vi "Autonomous Independent.vi"() -> ()   [LabVIEW 2015]
doc: "If AutoIDs match then TwoBall? is read from Dashboard, Else it is a control on the Front Panel\n\nINPUTS:\nTwoBall?\nState (Init)\nCollectorArmSpeed\nBrakeDistance\nSlowdownDistance\n\nSTATES:\n\nINIT: Clapper - In, SonicShifter Actuates to Low Gear, RollerPnuematic - Out, Servo - SetAngle (Indicator on Front Panel), IF TwoBall? == True: LowerArm ELSE CheckHotGoal\n\nCHECKHOTGOAL: Runs IsHotGoalDB and puts HotGoal? into Shift Register\n\nLOWERARM: Clapper - OUT, Wait = LowerArmTimeout / 2, RollerPneumatic - WAIT, Collector- LOWER\nWhen Collector has finished or after timeout from LowerArmTimeout and two other timers, Collector - STOP\nIF TwoBall? == TRUE then Collect ELSE Drive12ft\n\nPRECOLLECT: CollectorWrapper - PRECOLLECT\n\nDRIVEBACK: TankDrive -SETVALUE and DriveBackSpeed goes into both desired speeds, Wait - DriveBackWait, TankDrive - SETVALUE and 0 for both desired speeds\n\nCOLLECT: CollectWrapper - COLLECT\n\nSTOPCOLLECT: CollectWrapper - STOP\n\nLIFTARM: Collector - RAISE, Wait - LiftArmWait, Collector - STOP\n\nRAISESERVO: Servo - SETANGLE, Servo takes in RaiseServoAngle from Front Panel\n\nDRIVE12FT: Sonar - READVALUE, AutoDistance - LINEAR, Takes in Drive12ftDistance and distance from the Sonar and BrakeDistance and SlowdownDistance, TankDrive - LINEARDRIVE, Takes in both motor values from AutoDistance and MaxMotorChangeForward/Backward for Desired, TankDrive - LINEARDRIVE, Takes in 0 for Desired and MaxMotorChanges\n\nSHOOT12FT: IF not TwoBall? AND not HotGoal? then Wait - 5500 - ElapsedTime ELSE Pass, Wait - PreShootWait, ShooterWrapper - COLLECTORDOWN\n\nRAISEARM: Wait - PreRaiseArmWait, Collector - RAISE, Takes in CollectorArmSpeed, After Timeout from RaiseArmTimeout or Collector is done , Collector - STOP\n\nSHOOT3FT: Sonar - READVALUE, AutoDistance - LINEAR, Takes in Drive3ftDistance and output form Sonar and Brake/SlowdownDistance, TankDrive - SETVALUE, Takes in AutoDistance values for desired, Exits after AutoDistance is done or Drive3tfTimeout, TankDrive - SETVALUE, Takes in 0 for desired\n\nSHOOT3FT: ShooterWrapper - COLLECTORUP\n\nSTOP: Servo - SETANGLE, 0 for angle"
uses:
  AutoStates.ctl
  Robot Global Data.vi
  SingleSolenoidAction.ctl
  DoubleSolenoidAction.ctl
  ServoAction.ctl
  CollectorAction.ctl
  CollectorWrapAction.ctl
  TankDriveAction.ctl
  AutoAlignMode.ctl
  SonarAction.ctl
  ShooterWrapperAction.ctl
  AutoMode.ctl
  RollerAction.ctl
  LEDSaction.ctl
  HotGoalDetectType.ctl
panel:
  in  "PreScumbagWait":u32
  in  "HotGoalTypeDefault":T1
  out "KinectTriggered?":bool
  in  "EndInLowGear?":bool=TRUE
  in  "DriveBackWait":u32=1000
  in  "DriveBackSpeed":dbl=-1.0
  in  "PreCheckGoalWait":u32=260
  in  "BallSettleWait":u32=130
  in  "StartShootTime":u32=5000
  in  "StartInLowGear?":bool=TRUE
  in  "PreCollectWait":u32=400
  in  "AutoIDKey":i32=3061
  in  "DefaultMotorInput":dbl=1.0
  in  "DriveMinTime":u32=2000
  in  "RotateWait":u32=300
  in  "RotateMotorInput":dbl=0.7
  in  "DriveDistance":dbl=36.0 format="%#_13g"
  in  "DriveTimeout":u32=4000
  out "CheckGoalTimedOut?":bool
  in  "CheckHotGoalTimeout":u32=800
  in  "AutoDefaultMode":T2
  in  "ServoInitAngle":i32=140
  in  "RaiseServoAngle":i32=100
  in  "AccelBackward":dbl=0.1
  in  "PreRaiseArmWait":u32=500
  in  "AccelForward":dbl=0.1
  out "ElapsedTime":u32
  out "StateTime":u32
  out "CurrentState":T3
  out "RaiseArmTimedOut":bool
  out "Hot?":bool
  out "DriveTimeOut":bool
  out "LowerArmTimedOut":bool
  in  "RaiseArmTimeout":u32=800
  in  "SlowdownDistance":dbl=36.0 format="%#_13g"
  in  "BrakeDistance":dbl=12.0 format="%#_13g"
  in  "CollectorArmSpeed":dbl=1.0 format="%#_13g"
  in  "LiftArmWait":u32=200
  in  "PreDriveBackWait":u32
  in  "PreDriveBackSpeed":dbl
  in  "LowerArmTimeout":u32=800
  in  "error in":errorcluster
  out "error out":errorcluster
  # "SHOOT"
  # "SERVO"
  # "HOT GOAL"
  # "OUTPUT"
  # "ROTATE"
  # "GENERAL"
  # "DRIVE"
  # "RAISE/LOWER ARM"
  # "DEPRECATED"
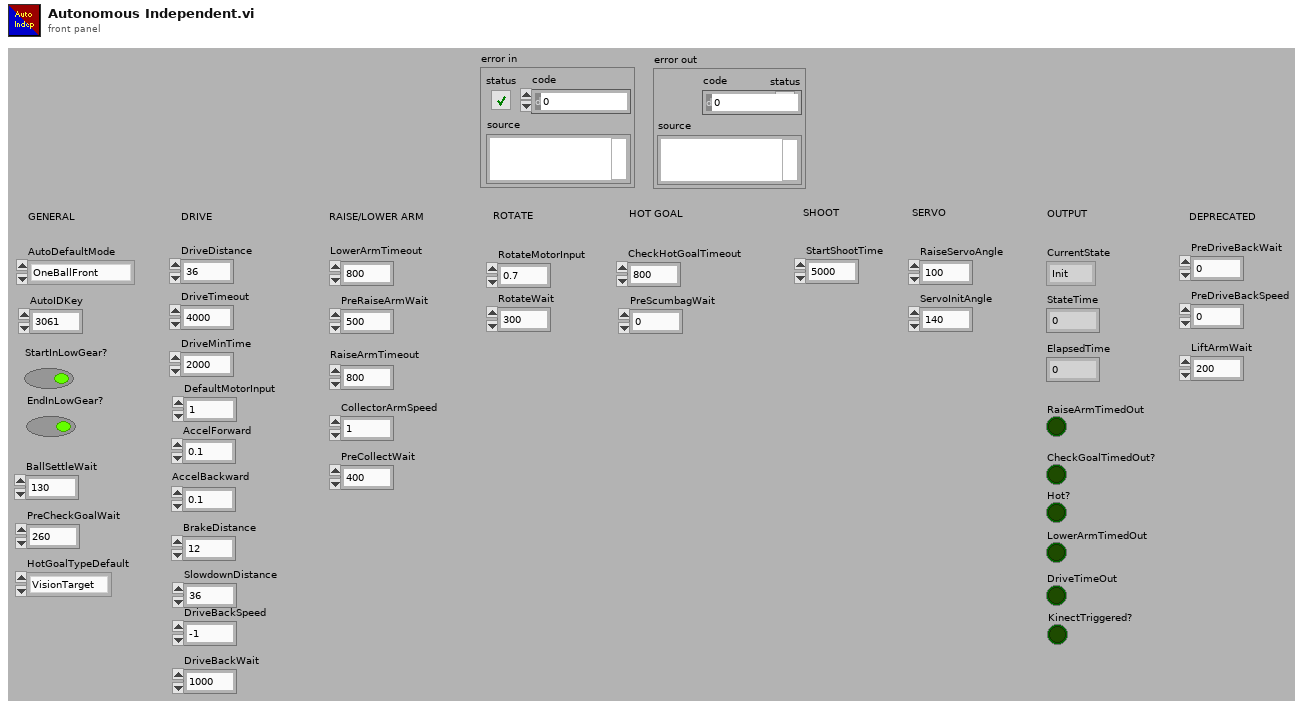
[diagram p1: front panel]
types:
  T1 = typedef "HotGoalDetectType.ctl" = enum16{"VisionTarget", "Kinect", "SoundDetect", "Webcam"}
  T2 = typedef "AutoMode.ctl" = enum16{"OneBallFront", "OneBallCollector", "TwoBallNormal", "TwoBallHot"}
  T3 = typedef "AutoStates.ctl" = enum16{"Init", "LowerArmCheckGoal", "DriveBack", "Collect", "StopCollect", "LiftArm", "RaiseServo", "Drive", "ShootCollectorUp", "RaiseArm", "ShootCollectorDown", "Rotate1", "Rotate2", "Stop"}
  T4 = typedef "SingleSolenoidAction.ctl" = enum16{"Init", "SetState", "Disable"}
  T5 = typedef "DoubleSolenoidAction.ctl" = enum16{"Init", "Middle", "In", "Out"}
  T6 = typedef "ServoAction.ctl" = enum16{"Init", "SetAngle", "GetAngle", "Lower", "Raise", "Disable"}
  T7 = typedef "CollectorAction.ctl" = enum16{"Init", "Raise", "Lower", "Stop", "GetStatus"}
  T8 = typedef "RollerAction.ctl" = enum16{"Init", "Off", "Forward", "Reverse"}
  T9 = typedef "TankDriveAction.ctl" = enum16{"Init", "LinearDrive", "SetValue", "Disable"}
  T10 = typedef "CollectorWrapAction.ctl" = enum16{"Stop", "PreCollect", "Collect"}
  T11 = typedef "AutoAlignMode.ctl" = enum16{"Fullspeed", "Linear"}
  T12 = typedef "SonarAction.ctl" = enum16{"Init", "ReadValue", "Disable"}
  T13 = typedef "LEDSaction.ctl" = enum16{"Init", "10SecondsLeft", "LimitDown", "LimitUp", "CollectDown", "CollectUp", "NotHot", "Hot", "Shift", "RollBack", "RollFwd", "Shoot", "Distance Low", "DistanceHigh", "PressureLow", "PressureHigh"}
  T14 = typedef "ShooterWrapperAction.ctl" = enum16{"Init", "CollectorDown", "CollectorUp"}
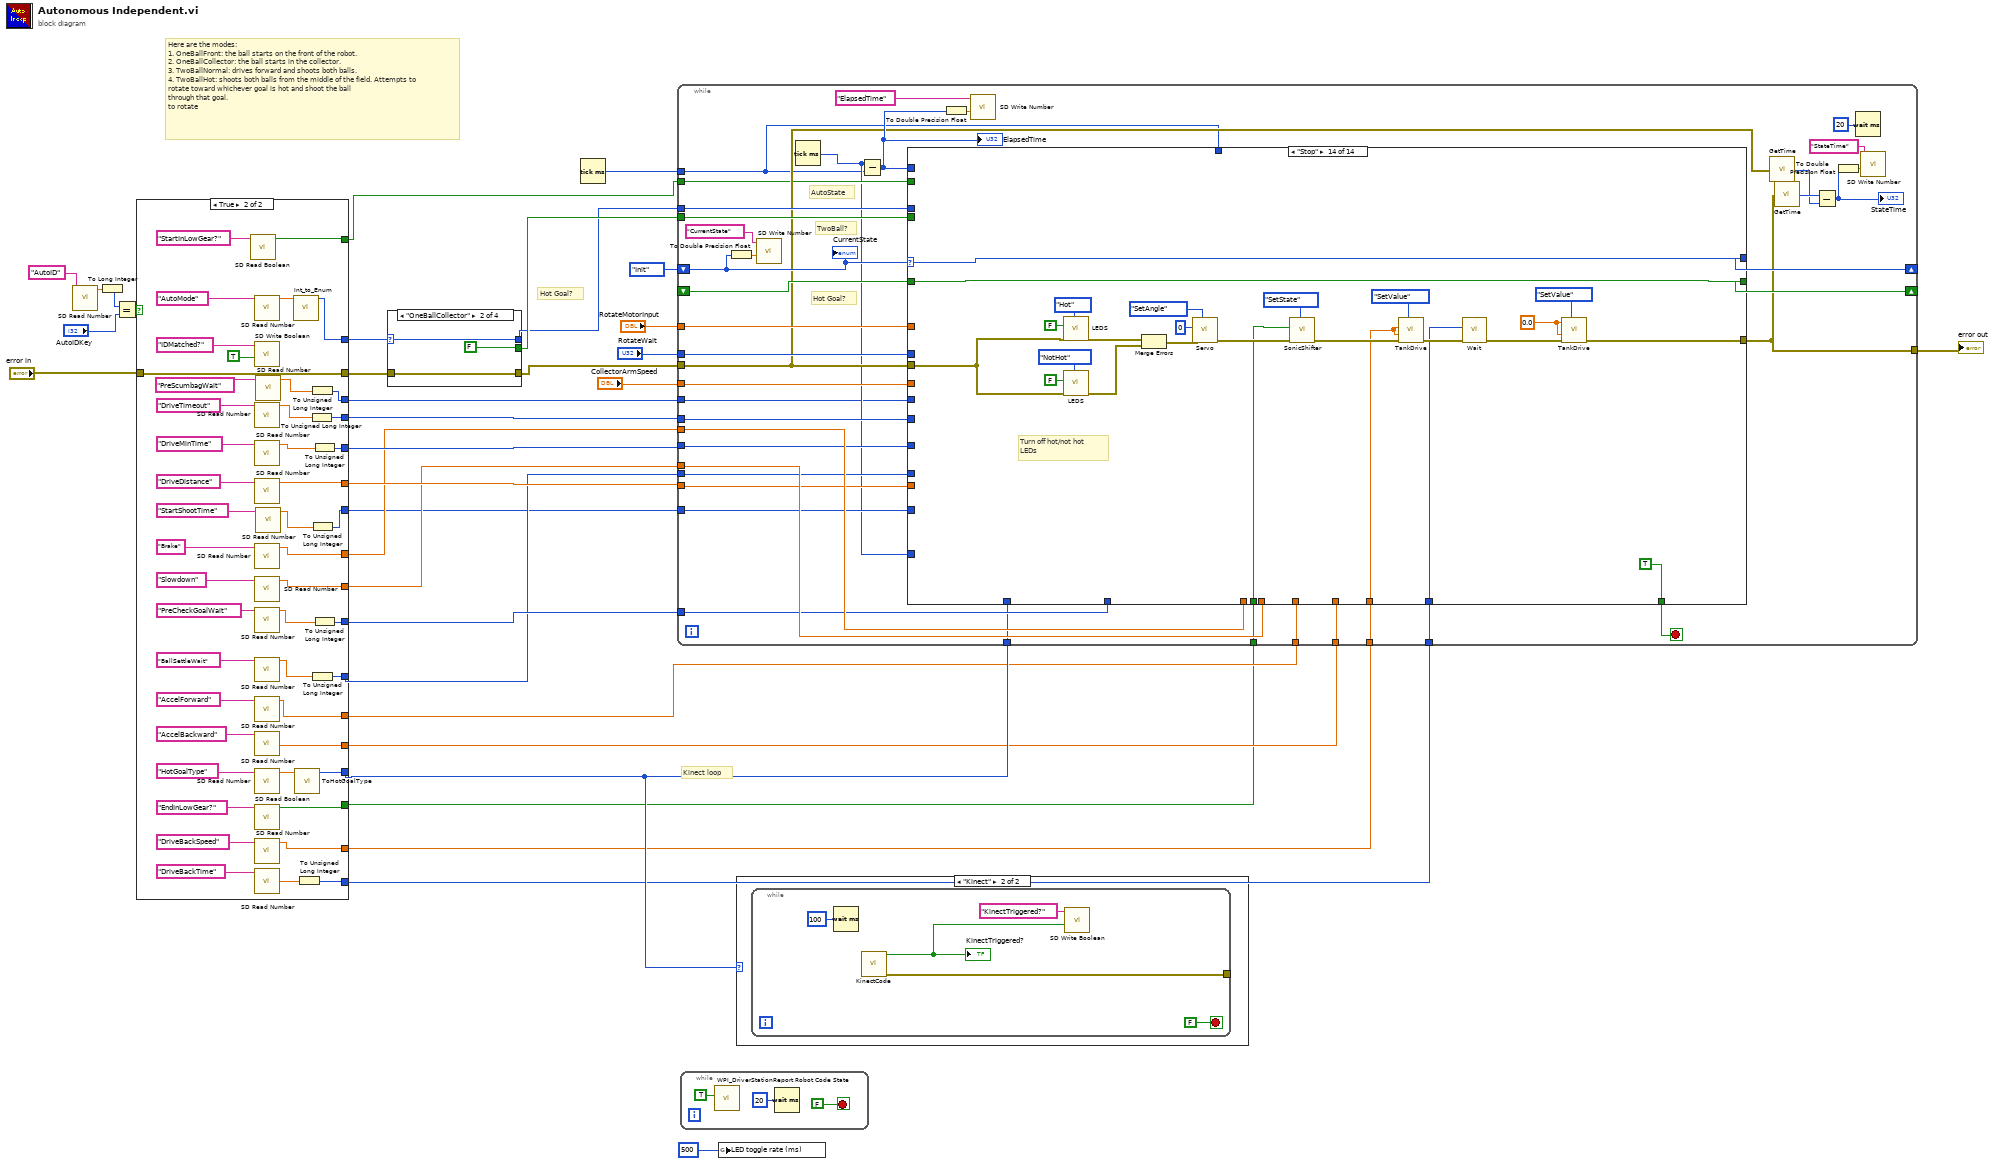
[diagram p0: block diagram]
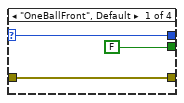
[diagram p3: hidden frame]
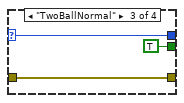
[diagram p4: hidden frame]
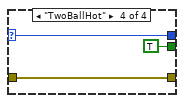
[diagram p5: hidden frame]
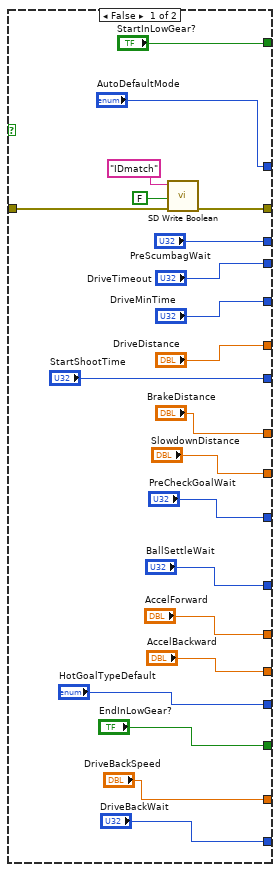
[diagram p6: hidden frame]
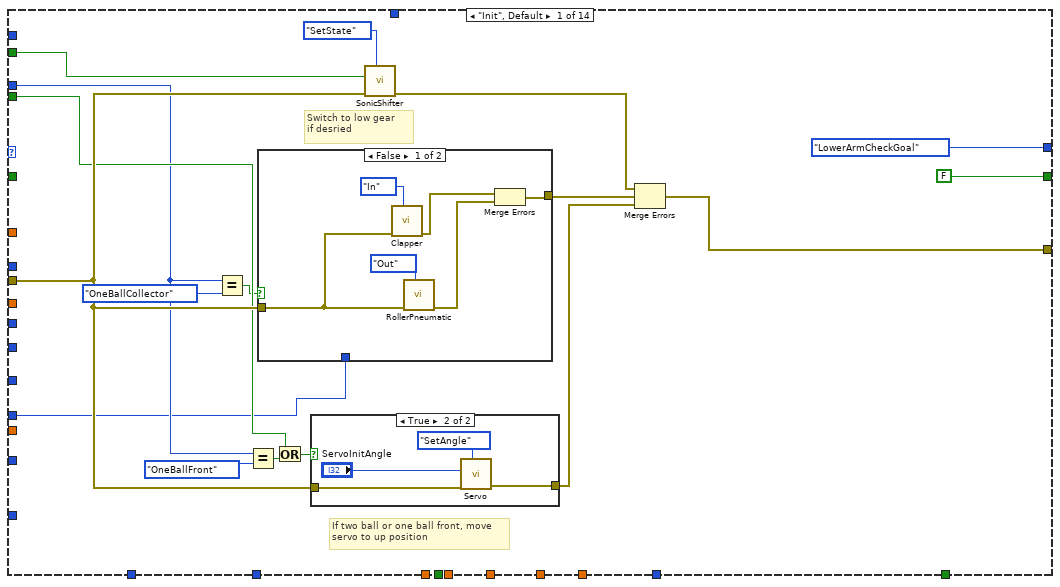
[diagram p7: hidden frame]
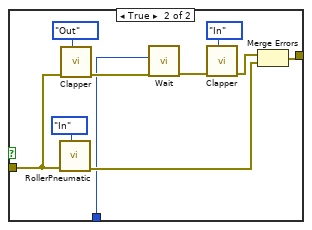
[diagram p8: hidden frame]
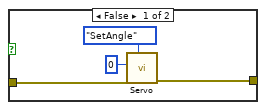
[diagram p9: hidden frame]
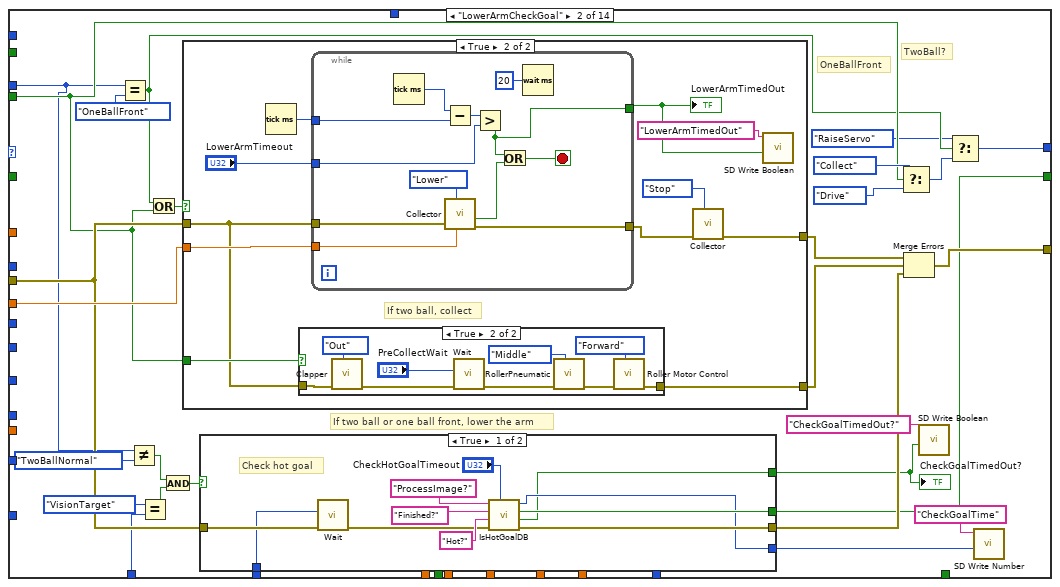
[diagram p10: hidden frame]
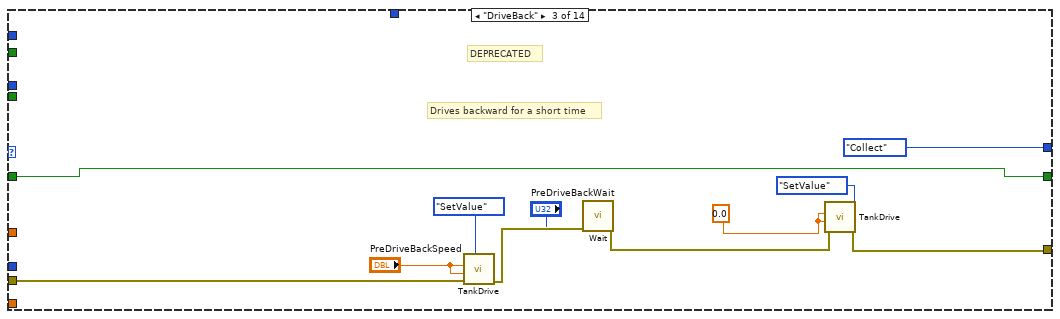
[diagram p14: hidden frame]
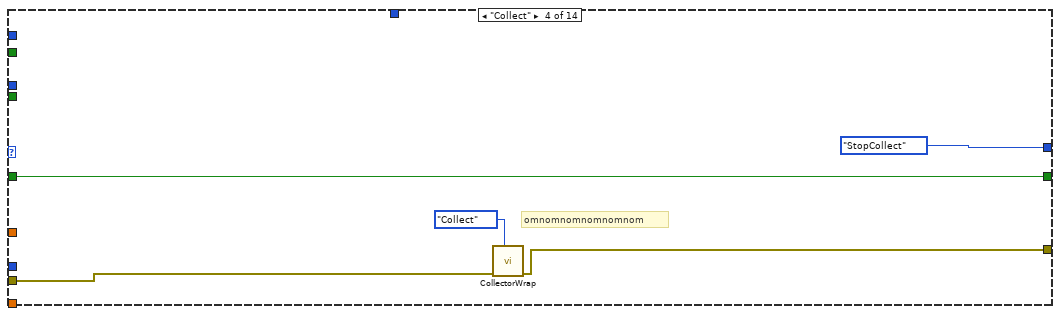
[diagram p15: hidden frame]
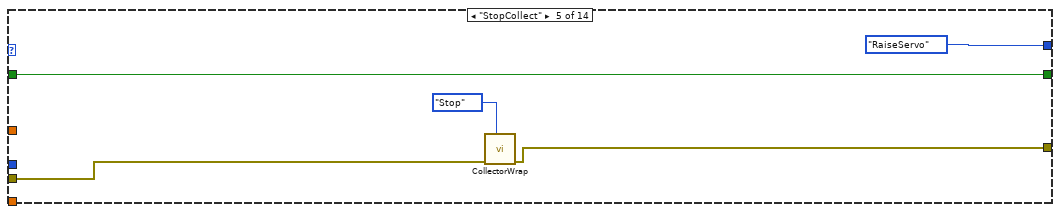
[diagram p16: hidden frame]
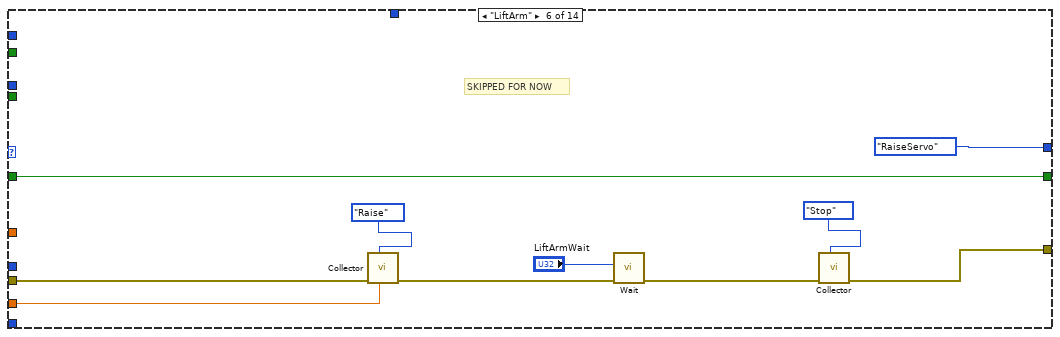
[diagram p17: hidden frame]
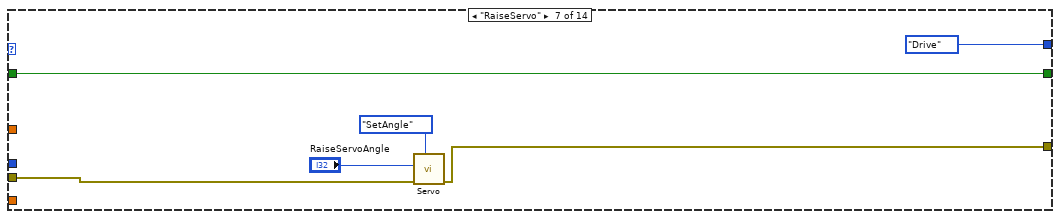
[diagram p18: hidden frame]
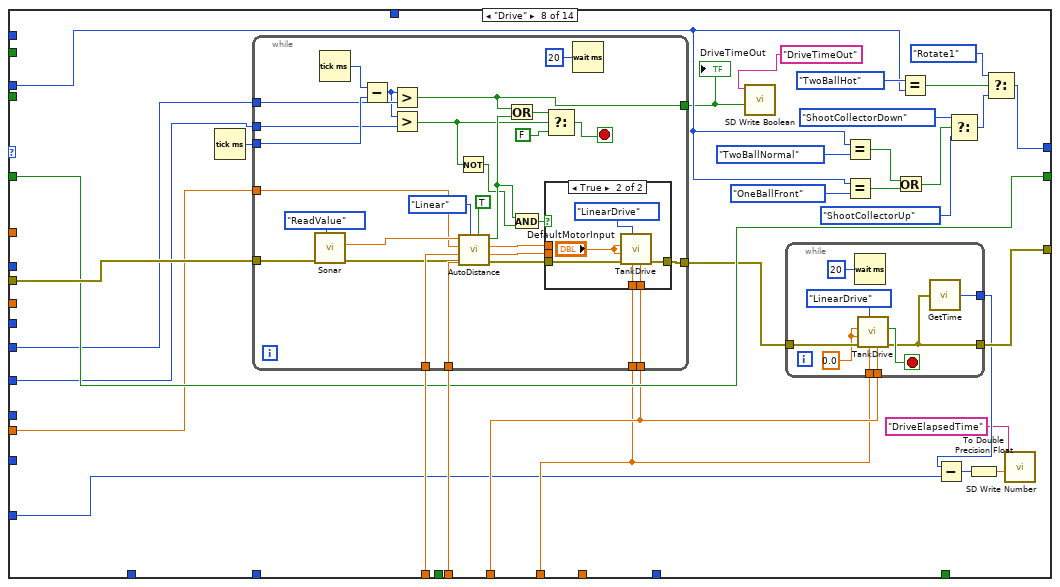
[diagram p19: hidden frame]
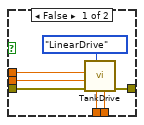
[diagram p20: hidden frame]
diagram:
  # "Kinect loop"
  # "Here are the modes:\n1. OneBallFront: the ball starts on the front of the robot.\n2. OneBallCollector: the ball starts in the collector.\n3. TwoBallNormal: drives forward and shoots both balls.\n4. TwoBallHot: shoots both balls from the middle of the field. Attempts to rotate toward whichever goal is hot and shoot the ball\nthrough that goal.\nto rotate"
  # "Hot Goal?"
  n1 = call <vilib>:"SD Read Number.vi"("Name"="AutoID") -> ("Numeric"=w33:dbl)  [unwired: 8 in, 2 out]
  n2 = To Long Integer(number=w33) -> (32bit integer=w19:i32)
  n3 = Equal?(x=w19, y="AutoIDKey") -> (x = y?=w28:bool)
  n4 = case shown="True" w28 {
    tunnel: "error in" -> [w54 w62]
    tunnel: [w53 w62] -> w24
    tunnel: ["AutoDefaultMode" w98] -> w26
    tunnel: ["DriveTimeout" w93] -> w14
    tunnel: ["DriveMinTime" w91] -> w15
    tunnel: ["DriveDistance" w89] -> w16
    tunnel: ["BrakeDistance" w87] -> w13
    tunnel: ["SlowdownDistance" w86] -> w12
    tunnel: ["PreCheckGoalWait" w83] -> w11
    tunnel: ["BallSettleWait" w80] -> w10
    tunnel: ["HotGoalTypeDefault" w76] -> w9
    tunnel: ["StartInLowGear?" w75] -> w8
    tunnel: ["AccelForward" w71] -> w7
    tunnel: ["AccelBackward" w70] -> w6
    tunnel: ["EndInLowGear?" w68] -> w5
    tunnel: ["DriveBackSpeed" w66] -> w4
    tunnel: ["DriveBackWait" w63] -> w3
    tunnel: ["StartShootTime" w59] -> w2
    tunnel: ["PreScumbagWait" w56] -> w1
    frame False {
      n5 = call <vilib>:"SD Write Boolean.vi"("error in"=w54, "Boolean"=FALSE, "Name"="IDmatch") -> ("error out"=w53:errorcluster)  [unwired: 7 in, 1 out]
    }
    frame True {
      n6 = call <vilib>:"SD Read Boolean.vi"("Name"="StartInLowGear?") -> ("Boolean"=w75:bool)  [unwired: 8 in, 2 out]
      n7 = call <vilib>:"SD Read Number.vi"("Name"="AutoMode") -> ("Numeric"=w99:dbl)  [unwired: 8 in, 2 out]
      n8 = call <vilib>:"SD Write Boolean.vi"("Boolean"=TRUE, "Name"="IDMatched?") -> ()  [unwired: 8 in, 2 out]
      n9 = call <vilib>:"SD Read Number.vi"("Name"="DriveTimeout") -> ("Numeric"=w92:dbl)  [unwired: 8 in, 2 out]
      n10 = call <vilib>:"SD Read Number.vi"("Name"="DriveMinTime") -> ("Numeric"=w90:dbl)  [unwired: 8 in, 2 out]
      n11 = call <vilib>:"SD Read Number.vi"("Name"="DriveDistance") -> ("Numeric"=w89:dbl)  [unwired: 8 in, 2 out]
      n12 = call <vilib>:"SD Read Number.vi"("Name"="Brake") -> ("Numeric"=w87:dbl)  [unwired: 8 in, 2 out]
      n13 = call <vilib>:"SD Read Number.vi"("Name"="Slowdown") -> ("Numeric"=w86:dbl)  [unwired: 8 in, 2 out]
      n14 = call <vilib>:"SD Read Number.vi"("Name"="PreCheckGoalWait") -> ("Numeric"=w82:dbl)  [unwired: 8 in, 2 out]
      n15 = call <vilib>:"SD Read Number.vi"("Name"="BallSettleWait") -> ("Numeric"=w79:dbl)  [unwired: 8 in, 2 out]
      n16 = call <vilib>:"SD Read Number.vi"("Name"="AccelForward") -> ("Numeric"=w71:dbl)  [unwired: 8 in, 2 out]
      n17 = call <vilib>:"SD Read Number.vi"("Name"="AccelBackward") -> ("Numeric"=w70:dbl)  [unwired: 8 in, 2 out]
      n18 = call <vilib>:"SD Read Number.vi"("Name"="HotGoalType") -> ("Numeric"=w77:dbl)  [unwired: 8 in, 2 out]
      n19 = call <vilib>:"SD Read Boolean.vi"("Name"="EndInLowGear?") -> ("Boolean"=w68:bool)  [unwired: 8 in, 2 out]
      n20 = call <vilib>:"SD Read Number.vi"("Name"="DriveBackSpeed") -> ("Numeric"=w66:dbl)  [unwired: 8 in, 2 out]
      n21 = call <vilib>:"SD Read Number.vi"("Name"="DriveBackTime") -> ("Numeric"=w65:dbl)  [unwired: 8 in, 2 out]
      n22 = call <vilib>:"SD Read Number.vi"("Name"="PreScumbagWait") -> ("Numeric"=w58:dbl)  [unwired: 8 in, 2 out]
      n23 = call <vilib>:"SD Read Number.vi"("Name"="StartShootTime") -> ("Numeric"=w61:dbl)  [unwired: 8 in, 2 out]
      n24 = call "Int_to_Enum.vi"("IntIn"=w99) -> ("EnumOut"=w98:T2)  [unwired: 10 in]
      n25 = call "ToHotGoalType.vi"("IntIn"=w77) -> ("EnumOut"=w76:T1)  [unwired: 10 in]
      n26 = To Unsigned Long Integer(number=w65) -> (unsigned 32bit integer=w63:u32)
      n27 = To Unsigned Long Integer(number=w92) -> (unsigned 32bit integer=w93:u32)
      n28 = To Unsigned Long Integer(number=w58) -> (unsigned 32bit integer=w56:u32)
      n29 = To Unsigned Long Integer(number=w79) -> (unsigned 32bit integer=w80:u32)
      n30 = To Unsigned Long Integer(number=w61) -> (unsigned 32bit integer=w59:u32)
      n31 = To Unsigned Long Integer(number=w90) -> (unsigned 32bit integer=w91:u32)
      n32 = To Unsigned Long Integer(number=w82) -> (unsigned 32bit integer=w83:u32)
    }
  }
  n33 = case shown="\"OneBallCollector\"" w26 {
    selector: w26 -> [w102 w105 w108 w111]
    tunnel: [FALSE FALSE TRUE TRUE] -> w25
    tunnel: w24 -> [w103 w106 w109 w112]
    tunnel: [w103 w106 w109 w112] -> w23
    tunnel: [w102 w105 w108 w111] -> w22
    frame "OneBallFront", Default {
    }
    frame "OneBallCollector" {
    }
    frame "TwoBallNormal" {
    }
    frame "TwoBallHot" {
    }
  }
  n34 = Tick Count (ms)() -> (millisecond timer value=w29:u32)
  n35 = while {
    shift-right: [w152] -> _
    shift-left: AutoStates."Init" ("Enum") -> [w134]
    shift-right: [w154] -> _
    shift-left: _ -> [w153]
    tunnel: w25 -> [w151]
    tunnel: "CollectorArmSpeed" -> [w149]
    tunnel: w13 -> [w147]
    tunnel: w12 -> [w148]
    tunnel: w29 -> [w114]
    tunnel: w23 -> [w131]
    tunnel: [w132] -> w34
    tunnel: w22 -> [w144]
    tunnel: "RotateMotorInput" -> [w143]
    tunnel: "RotateWait" -> [w142]
    tunnel: w2 -> [w129]
    tunnel: w16 -> [w128]
    tunnel: w15 -> [w127]
    tunnel: w14 -> [w126]
    tunnel: w11 -> [w125]
    tunnel: w10 -> [w124]
    tunnel: w9 -> [w123]
    tunnel: w8 -> [w122]
    tunnel: w7 -> [w121]
    tunnel: w6 -> [w120]
    tunnel: w5 -> [w118]
    tunnel: w4 -> [w117]
    tunnel: w3 -> [w116]
    tunnel: w1 -> [w115]
    stop <- w146 stop-if-true
    # "AutoState"
    # "TwoBall?"
    # "Hot Goal?"
    n36 = To Double Precision Float(number=w134) -> (double precision float=w135:dbl)
    n37 = call <vilib>:"SD Write Number.vi"("Numeric"=w135, "Name"="CurrentState") -> ()  [unwired: 8 in, 2 out]
    n38 = Tick Count (ms)() -> (millisecond timer value=w119:u32)
    n39 = Subtract(x=w119, y=w114) -> (x-y=w137:u32)
    "ElapsedTime" <- w137
    n40 = case shown="\"Stop\"" w134 {
      selector: w134 -> [_ _ _ _ _ _ _ _ _ _ _ _ _ w559]
      tunnel: w131 -> [w166 w221 w280 w285 w290 w295 w305 w337 w402 w465 w486 w509 w525 w541]
      tunnel: [w170 w220 w273 w284 w289 w294 w304 w334 w389 w463 w491 w504 w524 w547] -> w132
      tunnel: [FALSE ("Hot?") w208 w278 w282 w287 w293 w306 w326 w393 w464 w481 w507 w518 w560] -> w154
      tunnel: w153 -> [_ _ w278 w282 w287 w293 w306 w326 w408 w464 w481 w507 w518 w560]
      tunnel: [AutoStates."LowerArmCheckGoal" ("Enum") w209 AutoStates."Collect" ("Enum") AutoStates."StopCollect" ("Enum") AutoStates."RaiseServo" ("Enum") AutoStates."RaiseServo" ("Enum") AutoStates."Drive" ("Enum") w324 AutoStates."Stop" ("Enum") w449 AutoStates."RaiseArm" ("Enum") AutoStates."ShootCollectorDown" ("Enum") AutoStates."ShootCollectorUp" ("Enum") w559] -> w152
      tunnel: w151 -> [w162 w214 _ _ _ _ _ _ w417 w458 w484 _ _ _]
      tunnel: w149 -> [_ w222 _ _ _ w292 _ _ _ w466 _ _ _ _]
      tunnel: w148 -> [_ _ _ _ _ _ _ w336 _ _ _ _ _ _]
      tunnel: w147 -> [_ _ _ _ _ _ _ w335 _ _ _ _ _ _]
      tunnel: w137 -> [_ _ _ _ _ _ _ _ _ _ w483 _ _ _]
      tunnel: [_ _ _ _ _ _ _ _ _ _ _ _ _ TRUE] -> w146
      tunnel: w144 -> [w158 w197 _ _ _ _ _ w322 w411 w454 _ _ _ _]
      tunnel: w143 -> [_ _ _ _ _ _ _ _ _ _ _ w514 w527 _]
      tunnel: w142 -> [_ _ _ _ _ _ _ _ _ _ _ w506 w526 _]
      tunnel: w129 -> [_ _ _ _ _ _ _ _ w409 _ w480 _ _ _]
      tunnel: w128 -> [_ _ _ _ _ _ _ w316 _ _ _ _ _ _]
      tunnel: w127 -> [_ _ _ _ _ _ _ w315 _ _ _ _ _ _]
      tunnel: w126 -> [_ _ _ _ _ _ _ w314 _ _ _ _ _ _]
      tunnel: w125 -> [_ w207 _ _ _ _ _ _ _ _ _ _ _ _]
      tunnel: w124 -> [w156 _ _ _ _ _ _ _ _ _ _ _ _ _]
      tunnel: w123 -> [_ w202 _ _ _ _ _ _ w407 _ _ _ _ _]
      tunnel: w122 -> [w155 _ _ _ _ _ _ _ _ _ _ _ _ _]
      tunnel: w121 -> [_ _ _ _ _ _ _ w313 _ _ _ _ _ _]
      tunnel: w120 -> [_ _ _ _ _ _ _ w312 _ _ _ _ _ _]
      tunnel: w119 -> [_ _ _ _ _ _ _ w308 _ _ _ _ _ _]
      tunnel: w118 -> [_ _ _ _ _ _ _ _ _ _ _ _ _ w546]
      tunnel: w117 -> [_ _ _ _ _ _ _ _ _ _ _ _ _ w545]
      tunnel: w116 -> [_ _ _ _ _ _ _ _ _ _ _ _ _ w544]
      tunnel: w115 -> [_ _ _ _ _ _ _ _ w400 _ _ _ _ _]
      tunnel: w114 -> [_ _ _ _ _ _ _ _ w398 _ _ _ _ _]
      frame "Init", Default {
        # "If two ball or one ball front, move\nservo to up position"
        # "Switch to low gear\nif desried"
        n41 = Equal?(x=w158, y=AutoMode."OneBallCollector") -> (x = y?=w157:bool)
        n42 = Equal?(x=w158, y=AutoMode."OneBallFront") -> (x = y?=w161:bool)
        n43 = case shown="False" w157 {
          tunnel: [w175 w180] -> w171
          tunnel: w166 -> [w172 w185]
          tunnel: w156 -> [_ w178]
          frame False {
            n44 = call "Clapper.vi"("State"=DoubleSolenoidAction."In", "Error in"=w172) -> ("Error out"=w174:errorcluster)  [unwired: 9 in]
            n45 = call "RollerPneumatic.vi"("State"=DoubleSolenoidAction."Out", "Error in"=w172) -> ("Error out"=w173:errorcluster)  [unwired: 9 in]
            n46 = Merge Errors(w174, w173) -> (w175:errorcluster)
          }
          frame True {
            n47 = call "RollerPneumatic.vi"("State"=DoubleSolenoidAction."In", "Error in"=w185) -> ("Error out"=w181:errorcluster)  [unwired: 9 in]
            n48 = call "Clapper.vi"("State"=DoubleSolenoidAction."Out", "Error in"=w185) -> ("Error out"=w184:errorcluster)  [unwired: 9 in]
            n49 = call "Wait.vi"("error in"=w184, "milliseconds to wait"=w178) -> ("error out"=w183:errorcluster)  [unwired: 9 in]
            n50 = call "Clapper.vi"("State"=DoubleSolenoidAction."In", "Error in"=w183) -> ("Error out"=w182:errorcluster)  [unwired: 9 in]
            n51 = Merge Errors(w182, w181) -> (w180:errorcluster)
          }
        }
        n52 = Or(x=w162, y=w161) -> (x .or. y?=w163:bool)
        n53 = case shown="True" w163 {
          tunnel: w166 -> [w190 w195]
          tunnel: [w189 w194] -> w168
          frame False {
            n54 = call "Servo.vi"("Action"=ServoAction."SetAngle", "error in (no error)"=w190, "Angle (deg)"=0) -> ("error out"=w189:errorcluster)  [unwired: 7 in, 1 out]
          }
          frame True {
            n55 = call "Servo.vi"("Action"=ServoAction."SetAngle", "error in (no error)"=w195, "Angle (deg)"="ServoInitAngle") -> ("error out"=w194:errorcluster)  [unwired: 7 in, 1 out]
          }
        }
        n56 = call "SonicShifter.vi"("Action"=SingleSolenoidAction."SetState", "error in (no error)"=w166, "Actuate?"=w155) -> ("error out"=w167:errorcluster)  [unwired: 8 in]
        n57 = Merge Errors(w167, w171, w168) -> (w170:errorcluster)
      }
      frame "LowerArmCheckGoal" {
        # "If two ball or one ball front, lower the arm"
        # "OneBallFront"
        # "TwoBall?"
        n58 = Equal?(x=w197, y=AutoMode."OneBallFront") -> (x = y?=w212:bool)
        n59 = Not Equal?(x=w197, y=AutoMode."TwoBallNormal") -> (x != y?=w198:bool)
        n60 = Equal?(x=HotGoalDetectType."VisionTarget", y=w202) -> (x = y?=w200:bool)
        n61 = Or(x=w212, y=w214) -> (x .or. y?=w216:bool)
        n62 = And(x=w198, y=w200) -> (x .and. y?=w199:bool)
        n63 = case shown="True" w216 {
          tunnel: w222 -> [_ w246]
          tunnel: [w236 w245] -> w213
          tunnel: w221 -> [w236 w239]
          tunnel: [w236 w241] -> w217
          tunnel: w214 -> [_ w240]
          frame False {
          }
          frame True {
            # "If two ball, collect"
            n64 = Tick Count (ms)() -> (millisecond timer value=w247:u32)
            n65 = case shown="True" w240 {
              tunnel: [w248 w251] -> w241
              tunnel: w239 -> [w248 w252]
              frame False {
              }
              frame True {
                n66 = call "Clapper.vi"("State"=DoubleSolenoidAction."Out", "Error in"=w252) -> ("Error out"=w256:errorcluster)  [unwired: 9 in]
                n67 = call "Wait.vi"("error in"=w256, "milliseconds to wait"="PreCollectWait") -> ("error out"=w254:errorcluster)  [unwired: 9 in]
                n68 = call "RollerPneumatic.vi"("State"=DoubleSolenoidAction."Middle", "Error in"=w254) -> ("Error out"=w257:errorcluster)  [unwired: 9 in]
                n69 = call "Roller Motor Control.vi"("Action"=RollerAction."Forward", "Error in"=w257) -> ("Error out"=w251:errorcluster)  [unwired: 9 in]
              }
            }
            n70 = while {
              tunnel: w239 -> [w258]
              tunnel: [w269] -> w242
              tunnel: w247 -> [w262]
              tunnel: w246 -> [w261]
              tunnel: [w260] -> w238
              tunnel: "LowerArmTimeout" -> [w259]
              stop <- w264 stop-if-true
              n71 = Tick Count (ms)() -> (millisecond timer value=w266:u32)
              n72 = Subtract(x=w266, y=w262) -> (x-y=w267:u32)
              n73 = call "Collector.vi"("MotorSpeed"=w261, "Action"=CollectorAction."Lower", "Error in"=w258) -> ("Error out"=w269:errorcluster, "Lower Triggered?"=w263:bool)  [unwired: 6 in, 1 out]
              n74 = Greater?(x=w267, y=w259) -> (0:w260:bool)
              n75 = Or(x=w260, y=w263) -> (x .or. y?=w264:bool)
              n76 = Wait (ms)(milliseconds to wait=u32 20) -> ()  [unwired: 1 out]
            }
            "LowerArmTimedOut" <- w238
            n77 = call "Collector.vi"("Action"=CollectorAction."Stop", "Error in"=w242) -> ("Error out"=w245:errorcluster)  [unwired: 7 in, 2 out]
            n78 = call <vilib>:"SD Write Boolean.vi"("Boolean"=w238, "Name"="LowerArmTimedOut") -> ()  [unwired: 8 in, 2 out]
          }
        }
        n79 = case shown="True" w199 {
          tunnel: w221 -> [w230 w235]
          tunnel: [w229 w235] -> w219
          tunnel: [w226 _] -> w208
          tunnel: w207 -> [w227 _]
          tunnel: [w225 _] -> w204
          tunnel: [w224 _] -> w203
          frame True {
            # "Check hot goal"
            n80 = call "Wait.vi"("error in"=w230, "milliseconds to wait"=w227) -> ("error out"=w228:errorcluster)  [unwired: 9 in]
            n81 = call "IsHotGoalDB.vi"("Timeout (ms)"="CheckHotGoalTimeout", "error in"=w228, "DBHot?"="Hot?", "DBFinished?"="Finished?", "DBStart"="ProcessImage?") -> ("error out"=w229:errorcluster, "TimedOut?"=w224:bool, "Hot?"=w226:bool, "ElapsedTime"=w225:u32)  [unwired: 3 in]
          }
          frame False {
          }
        }
        "CheckGoalTimedOut?" <- w203
        n82 = Select(t=AutoStates."Collect" ("Enum"), s=w214, f=AutoStates."Drive" ("Enum")) -> (s? t:f=w210:T3)
        n83 = Merge Errors(w213, w217, w219) -> (w220:errorcluster)
        n84 = call <vilib>:"SD Write Boolean.vi"("Boolean"=w203, "Name"="CheckGoalTimedOut?") -> ()  [unwired: 8 in, 2 out]
        n85 = Select(t=AutoStates."RaiseServo" ("Enum"), s=w212, f=w210) -> (s? t:f=w209:T3)
        n86 = call <vilib>:"SD Write Number.vi"("Numeric"=w204, "Name"="CheckGoalTime") -> ()  [unwired: 8 in, 2 out]
      }
      frame "DriveBack" {
        w271 = 0.0 ("LeftDesired")
        # "Drives backward for a short time"
        # "DEPRECATED"
        n87 = call "TankDrive.vi"("DriveAction"=TankDriveAction."SetValue", "error in (no error)"=w280, "RightDesired"="PreDriveBackSpeed", "LeftDesired"="PreDriveBackSpeed") -> ("error out"=w279:errorcluster)  [unwired: 6 in, 1 out]
        n88 = call "Wait.vi"("error in"=w279, "milliseconds to wait"="PreDriveBackWait") -> ("error out"=w274:errorcluster)  [unwired: 9 in]
        n89 = call "TankDrive.vi"("DriveAction"=TankDriveAction."SetValue", "error in (no error)"=w274, "RightDesired"=w271, "LeftDesired"=w271) -> ("error out"=w273:errorcluster)  [unwired: 6 in, 1 out]
      }
      frame "Collect" {
        # "omnomnomnomnomnom"
        n90 = call "CollectorWrap.vi"("Action"=CollectorWrapAction."Collect", "error in"=w285) -> ("error out"=w284:errorcluster)  [unwired: 9 in]
      }
      frame "StopCollect" {
        n91 = call "CollectorWrap.vi"("Action"=CollectorWrapAction."Stop", "error in"=w290) -> ("error out"=w289:errorcluster)  [unwired: 9 in]
      }
      frame "LiftArm" {
        # "SKIPPED FOR NOW"
        n92 = call "Collector.vi"("MotorSpeed"=w292, "Action"=CollectorAction."Raise" ("CollectorAction"), "Error in"=w295) -> ("Error out"=w296:errorcluster)  [unwired: 6 in, 2 out]
        n93 = call "Wait.vi"("error in"=w296, "milliseconds to wait"="LiftArmWait") -> ("error out"=w297:errorcluster)  [unwired: 9 in]
        n94 = call "Collector.vi"("Action"=CollectorAction."Stop" ("CollectorAction"), "Error in"=w297) -> ("Error out"=w294:errorcluster)  [unwired: 7 in, 2 out]
      }
      frame "RaiseServo" {
        n95 = call "Servo.vi"("Action"=ServoAction."SetAngle", "error in (no error)"=w305, "Angle (deg)"="RaiseServoAngle") -> ("error out"=w304:errorcluster)  [unwired: 7 in, 1 out]
      }
      frame "Drive" {
        n96 = Tick Count (ms)() -> (millisecond timer value=w338:u32)
        n97 = while {
          tunnel: w337 -> [w368]
          tunnel: [w372] -> w319
          tunnel: w338 -> [w373]
          tunnel: w336 -> [w370]
          tunnel: w335 -> [w371]
          tunnel: [w355] -> w318
          tunnel: w313 -> [w364]
          tunnel: w312 -> [w363]
          tunnel: w314 -> [w362]
          tunnel: w316 -> [w361]
          tunnel: w315 -> [w356]
          stop <- w353 stop-if-true
          n98 = call "Sonar.vi"("Action"=SonarAction."ReadValue", "error in (no error)"=w368) -> ("error out"=w365:errorcluster, "distance"=w367:dbl)  [unwired: 8 in]
          n99 = Tick Count (ms)() -> (millisecond timer value=w374:u32)
          n100 = Subtract(x=w374, y=w373) -> (x-y=w357:u32)
          n101 = Greater?(x=w357, y=w362) -> (0:w355:bool)
          n102 = Greater?(x=w357, y=w356) -> (0:w350:bool)
          n103 = Not(x=w350) -> (.not. x?=w349:bool)
          n104 = call "AutoDistance.vi"("Auto"=TRUE, "Mode"=AutoAlignMode."Linear", "Slowdown"=w370, "Brake"=w371, "DesiredDistance"=w361, "CurrentDistance"=w367) -> ("TankDriveRight"=w359:dbl, "TankDriveLeft"=w358:dbl, "Finished"=w351:bool)  [unwired: 3 in]
          n105 = Or(x=w355, y=w351) -> (x .or. y?=w354:bool)
          n106 = And(x=w351, y=w349) -> (x .and. y?=w352:bool)
          n107 = case shown="True" w352 {
            tunnel: [w381 w387] -> w372
            tunnel: w365 -> [w380 w386]
            tunnel: w364 -> [w376 w385]
            tunnel: w363 -> [w377 w384]
            tunnel: w359 -> [w378 _]
            tunnel: w358 -> [w379 _]
            frame False {
              n108 = call "TankDrive.vi"("MaxMotorChangeForward"=w376, "MaxMotorChangeBackwrad"=w377, "DriveAction"=TankDriveAction."LinearDrive", "error in (no error)"=w380, "RightDesired"=w378, "LeftDesired"=w379) -> ("error out"=w381:errorcluster)  [unwired: 4 in, 1 out]
            }
            frame True {
              n109 = call "TankDrive.vi"("MaxMotorChangeForward"=w385, "MaxMotorChangeBackwrad"=w384, "DriveAction"=TankDriveAction."LinearDrive", "error in (no error)"=w386, "RightDesired"="DefaultMotorInput", "LeftDesired"="DefaultMotorInput") -> ("error out"=w387:errorcluster)  [unwired: 4 in, 1 out]
            }
          }
          n110 = Select(t=w354, s=w350, f=FALSE) -> (s? t:f=w353:bool)
          n111 = Wait (ms)(milliseconds to wait=u32 20) -> ()  [unwired: 1 out]
        }
        "DriveTimeOut" <- w318
        n112 = call <vilib>:"SD Write Boolean.vi"("Boolean"=w318, "Name"="DriveTimeOut") -> ()  [unwired: 8 in, 2 out]
        n113 = while {
          tunnel: w319 -> [w347]
          tunnel: [w339] -> w334
          tunnel: w313 -> [w342]
          tunnel: w312 -> [w341]
          tunnel: [w340] -> w309
          stop <- w343 stop-if-true
          w346 = 0.0 ("LeftDesired")
          n114 = Wait (ms)(milliseconds to wait=u32 20) -> ()  [unwired: 1 out]
          n115 = call "TankDrive.vi"("MaxMotorChangeForward"=w342, "MaxMotorChangeBackwrad"=w341, "DriveAction"=TankDriveAction."LinearDrive", "error in (no error)"=w347, "RightDesired"=w346, "LeftDesired"=w346) -> ("error out"=w339:errorcluster, "InRange?"=w343:bool)  [unwired: 4 in]
          n116 = call "GetTime.vi"("error in"=w339) -> ("Time"=w340:u32)
        }
        n117 = Equal?(x=w322, y=AutoMode."TwoBallNormal") -> (x = y?=w332:bool)
        n118 = Equal?(x=w322, y=AutoMode."OneBallFront") -> (x = y?=w331:bool)
        n119 = Or(x=w332, y=w331) -> (x .or. y?=w327:bool)
        n120 = Equal?(x=AutoMode."TwoBallHot" ("y"), y=w322) -> (x = y?=w321:bool)
        n121 = Subtract(x=w309, y=w308) -> (x-y=w310:u32)
        n122 = Select(t=AutoStates."ShootCollectorDown" ("Enum"), s=w327, f=AutoStates."ShootCollectorUp") -> (s? t:f=w325:T3)
        n123 = To Double Precision Float(number=w310) -> (double precision float=w311:dbl)
        n124 = Select(t=AutoStates."Rotate1" ("Enum"), s=w321, f=w325) -> (s? t:f=w324:T3)
        n125 = call <vilib>:"SD Write Number.vi"("Numeric"=w311, "Name"="DriveElapsedTime") -> ()  [unwired: 8 in, 2 out]
      }
      frame "ShootCollectorUp" {
        # "Set LEDS to\ncorrect state\nfor hot/not"
        n126 = call "Wait.vi"("error in"=w402, "milliseconds to wait"=w400) -> ("error out"=w401:errorcluster)  [unwired: 9 in]
        n127 = case shown="\"VisionTarget\", Default" w407 {
          tunnel: w408 -> [w421 _ _ _]
          tunnel: [w421 w423 w426 w429] -> w393
          tunnel: w401 -> [w420 w422 w425 w432]
          tunnel: [w420 w422 w425 w432] -> w397
          frame "VisionTarget", Default {
          }
          frame "Kinect" {
            n128 = local read "KinectTriggered?"() -> (w424:bool)
            n129 = Not(x=w424) -> (.not. x?=w423:bool)
          }
          frame "SoundDetect" {
            n130 = call <vilib>:"SD Read Boolean.vi"("Name"="PitchDetected") -> ("Boolean"=w428:bool)  [unwired: 8 in, 2 out]
            n131 = Not(x=w428) -> (.not. x?=w426:bool)
          }
          frame "Webcam" {
            n132 = call <vilib>:"SD Read Boolean.vi"("Name"="WebcamMatched?") -> ("Boolean"=w431:bool)  [unwired: 8 in, 2 out]
            n133 = Not(x=w431) -> (.not. x?=w429:bool)
          }
        }
        "Hot?" <- w393
        n134 = Not(x=w393) -> (.not. x?=w416:bool)
        n135 = Not(x=w417) -> (.not. x?=w418:bool)
        n136 = And(x=w418, y=w416) -> (x .and. y?=w414:bool)
        n137 = Equal?(x=w411, y=AutoMode."TwoBallHot") -> (x = y?=w412:bool)
        n138 = Or(x=w414, y=w412) -> (x .or. y?=w413:bool)
        n139 = case shown="True" w413 {
          tunnel: w397 -> [w434 w438]
          tunnel: [w434 w440] -> w403
          tunnel: w409 -> [_ w442]
          tunnel: [w433 w439] -> w399
          tunnel: w398 -> [_ w436]
          frame False {
            n140 = call "GetTime.vi"("error in"=w434) -> ("Time"=w433:u32)
          }
          frame True {
            n141 = call "GetTime.vi"("error in"=w438) -> ("Time"=w437:u32)
            n142 = Subtract(x=w437, y=w436) -> (x-y=w435:u32)
            n143 = Subtract(x=w442, y=w435) -> (x-y=w443:u32)
            n144 = Greater?(x=w442, y=w435) -> (0:w444:bool)
            n145 = case shown="False" w444 {
              tunnel: [u32 0 w446] -> w441
              tunnel: w443 -> [_ w446]
              frame False {
              }
              frame True {
              }
            }
            n146 = call "Wait.vi"("error in"=w438, "milliseconds to wait"=w441) -> ("error out"=w440:errorcluster)  [unwired: 9 in]
            n147 = call "GetTime.vi"("error in"=w440) -> ("Time"=w439:u32)
          }
        }
        n148 = call <vilib>:"SD Write Boolean.vi"("Boolean"=w393, "Name"="WasHot?") -> ()  [unwired: 8 in, 2 out]
        n149 = Not(x=w393) -> (.not. x?=w394:bool)
        n150 = call "LEDS.vi"("Action"=LEDSaction."Hot", "error in"=w397, "On/Off"=w393) -> ("error out"=w391:errorcluster)  [unwired: 8 in]
        n151 = call "LEDS.vi"("Action"=LEDSaction."NotHot", "error in"=w397, "On/Off"=w394) -> ("error out"=w390:errorcluster)  [unwired: 8 in]
        n152 = Subtract(x=w399, y=w398) -> (x-y=w404:u32)
        n153 = call "ShooterWrapper.vi"("Action"=ShooterWrapperAction."CollectorUp", "error in"=w403) -> ("error out"=w392:errorcluster)  [unwired: 8 in]
        n154 = call <vilib>:"SD Write Number.vi"("Numeric"=w404, "Name"="ShootTime") -> ()  [unwired: 8 in, 2 out]
        n155 = Merge Errors(w392, w391, w390) -> (w389:errorcluster)
      }
      frame "RaiseArm" {
        # "Hot Goal?"
        # "TwoBall?"
        # "Give shooter\ntime to come back down"
        n156 = call "Wait.vi"("error in"=w465, "milliseconds to wait"="PreRaiseArmWait") -> ("error out"=w461:errorcluster)  [unwired: 9 in]
        n157 = Tick Count (ms)() -> (millisecond timer value=w467:u32)
        n158 = while {
          tunnel: w461 -> [w479]
          tunnel: [w478] -> w459
          tunnel: w467 -> [w471]
          tunnel: w466 -> [w470]
          tunnel: [w469] -> w448
          stop <- w472 stop-if-true
          n159 = Tick Count (ms)() -> (millisecond timer value=w474:u32)
          n160 = Subtract(x=w474, y=w471) -> (x-y=w475:u32)
          n161 = call "Collector.vi"("MotorSpeed"=w470, "Action"=CollectorAction."Raise", "Error in"=w479) -> ("Error out"=w478:errorcluster, "Upper Triggered?"=w468:bool)  [unwired: 6 in, 1 out]
          n162 = Greater?(x=w475, y="RaiseArmTimeout") -> (0:w469:bool)
          n163 = Wait (ms)(milliseconds to wait=u32 20) -> ()  [unwired: 1 out]
          n164 = Or(x=w469, y=w468) -> (x .or. y?=w472:bool)
        }
        "RaiseArmTimedOut" <- w448
        n165 = call "Collector.vi"("Action"=CollectorAction."Stop", "Error in"=w459) -> ("Error out"=w463:errorcluster)  [unwired: 7 in, 2 out]
        n166 = call <vilib>:"SD Write Boolean.vi"("Boolean"=w448, "Name"="RaiseArmTimedOut") -> ()  [unwired: 8 in, 2 out]
        n167 = Equal?(x=w454, y=AutoMode."TwoBallHot") -> (x = y?=w452:bool)
        n168 = Not(x=w458) -> (.not. x?=w457:bool)
        n169 = Select(t=AutoStates."Stop" ("Enum"), s=w457, f=AutoStates."ShootCollectorUp" ("Enum")) -> (s? t:f=w450:T3)
        n170 = Select(t=AutoStates."Rotate2" ("Enum"), s=w452, f=w450) -> (s? t:f=w449:T3)
      }
      frame "ShootCollectorDown" {
        # "AND"
        # "001\n111\n010\n100"
        n171 = Not(x=w484) -> (.not. x?=w488:bool)
        n172 = Not(x=w481) -> (.not. x?=w487:bool)
        n173 = And(x=w488, y=w487) -> (x .and. y?=w482:bool)
        n174 = case shown="True" w482 {
          tunnel: w486 -> [w492 w499]
          tunnel: [w492 w498] -> w485
          tunnel: w483 -> [_ w497]
          tunnel: w480 -> [_ w493]
          frame False {
          }
          frame True {
            n175 = Subtract(x=w493, y=w497) -> (x-y=w494:u32)
            n176 = Greater?(x=w493, y=w497) -> (0:w496:bool)
            n177 = case shown="False" w496 {
              tunnel: [u32 0 w501] -> w495
              tunnel: w494 -> [_ w501]
              frame False {
              }
              frame True {
              }
            }
            n178 = call "Wait.vi"("error in"=w499, "milliseconds to wait"=w495) -> ("error out"=w498:errorcluster)  [unwired: 9 in]
          }
        }
        n179 = call "ShooterWrapper.vi"("Action"=ShooterWrapperAction."CollectorDown", "error in"=w485) -> ("error out"=w491:errorcluster)  [unwired: 8 in]
      }
      frame "Rotate1" {
        w503 = 0.0
        # "ASSUME CAMERA POINTED LEFT"
        n180 = Select(t=1.0, s=w507, f=-1.0) -> (s? t:f=w516:dbl)
        n181 = Multiply(x=w516, y=w514) -> (x*y=w513:dbl)
        n182 = Negate(x=w513) -> (-x=w512:dbl)
        n183 = call "TankDrive.vi"("DriveAction"=TankDriveAction."SetValue", "error in (no error)"=w509, "RightDesired"=w513, "LeftDesired"=w512) -> ("error out"=w508:errorcluster)  [unwired: 6 in, 1 out]
        n184 = call "Wait.vi"("error in"=w508, "milliseconds to wait"=w506) -> ("error out"=w505:errorcluster)  [unwired: 9 in]
        n185 = call "TankDrive.vi"("DriveAction"=TankDriveAction."SetValue", "error in (no error)"=w505, "RightDesired"=w503, "LeftDesired"=w503) -> ("error out"=w504:errorcluster)  [unwired: 6 in, 1 out]
      }
      frame "Rotate2" {
        w529 = 0.0
        n186 = Select(t=1.0, s=w518, f=-1.0) -> (s? t:f=w534:dbl)
        n187 = Multiply(x=w534, y=w527) -> (x*y=w523:dbl)
        n188 = Negate(x=w523) -> (-x=w522:dbl)
        n189 = call "TankDrive.vi"("DriveAction"=TankDriveAction."SetValue", "error in (no error)"=w525, "RightDesired"=w522, "LeftDesired"=w523) -> ("error out"=w531:errorcluster)  [unwired: 6 in, 1 out]
        n190 = Multiply(x=u32 2, y=w526) -> (x*y=w521:u32)
        n191 = call "Wait.vi"("error in"=w531, "milliseconds to wait"=w521) -> ("error out"=w530:errorcluster)  [unwired: 9 in]
        n192 = call "TankDrive.vi"("DriveAction"=TankDriveAction."SetValue", "error in (no error)"=w530, "RightDesired"=w529, "LeftDesired"=w529) -> ("error out"=w524:errorcluster)  [unwired: 6 in, 1 out]
      }
      frame "Stop" {
        w551 = 0.0 ("LeftDesired")
        # "Turn off hot/not hot\nLEDs"
        n193 = call "LEDS.vi"("Action"=LEDSaction."Hot", "error in"=w541, "On/Off"=FALSE) -> ("error out"=w538:errorcluster)  [unwired: 8 in]
        n194 = call "LEDS.vi"("Action"=LEDSaction."NotHot", "error in"=w541, "On/Off"=FALSE) -> ("error out"=w537:errorcluster)  [unwired: 8 in]
        n195 = Merge Errors(w538, w537) -> (w536:errorcluster)
        n196 = call "Servo.vi"("Action"=ServoAction."SetAngle", "error in (no error)"=w536, "Angle (deg)"=0) -> ("error out"=w549:errorcluster)  [unwired: 7 in, 1 out]
        n197 = call "SonicShifter.vi"("Action"=SingleSolenoidAction."SetState", "error in (no error)"=w549, "Actuate?"=w546) -> ("error out"=w548:errorcluster)  [unwired: 8 in]
        n198 = call "TankDrive.vi"("DriveAction"=TankDriveAction."SetValue", "error in (no error)"=w548, "RightDesired"=w545, "LeftDesired"=w545) -> ("error out"=w553:errorcluster)  [unwired: 6 in, 1 out]
        n199 = call "Wait.vi"("error in"=w553, "milliseconds to wait"=w544) -> ("error out"=w552:errorcluster)  [unwired: 9 in]
        n200 = call "TankDrive.vi"("DriveAction"=TankDriveAction."SetValue", "error in (no error)"=w552, "RightDesired"=w551, "LeftDesired"=w551) -> ("error out"=w547:errorcluster)  [unwired: 6 in, 1 out]
      }
    }
    n201 = To Double Precision Float(number=w137) -> (double precision float=w136:dbl)
    n202 = call <vilib>:"SD Write Number.vi"("Numeric"=w136, "Name"="ElapsedTime") -> ()  [unwired: 8 in, 2 out]
    n203 = call "GetTime.vi"("error in"=w131) -> ("Time"=w130:u32)
    n204 = call "GetTime.vi"("error in"=w132) -> ("Time"=w145:u32)
    n205 = Subtract(x=w145, y=w130) -> (x-y=w141:u32)
    "StateTime" <- w141
    n206 = To Double Precision Float(number=w141) -> (double precision float=w139:dbl)
    n207 = Wait (ms)(milliseconds to wait=u32 20) -> ()  [unwired: 1 out]
    n208 = call <vilib>:"SD Write Number.vi"("Numeric"=w139, "Name"="StateTime") -> ()  [unwired: 8 in, 2 out]
    "CurrentState" <- w134
  }
  "error out" <- w34
  n209 = while {
    stop <- FALSE stop-if-true
    n210 = call <vilib>:"WPI_DriverStationReport Robot Code State.vi"("Autonomous"=TRUE) -> ()  [unwired: 10 in, 1 out]
    n211 = Wait (ms)(milliseconds to wait=u32 20) -> ()  [unwired: 1 out]
  }
  n212 = global write "Robot Global Data.vi" "LED toggle rate (ms)"(u32 500 ("LED ms toggle rate")) -> ()
  n213 = case shown="\"Kinect\"" w9 {
    frame "VisionTarget", Default {
    }
    frame "Kinect" {
      n214 = while {
        tunnel: [w566] -> _
        stop <- FALSE stop-if-true
        n215 = Wait (ms)(milliseconds to wait=u32 100) -> ()  [unwired: 1 out]
        n216 = call "KinectCode.vi"() -> ("error out"=w566:errorcluster, "HandsApart?"=w565:bool)  [unwired: 10 in]
        "KinectTriggered?" <- w565
        n217 = call <vilib>:"SD Write Boolean.vi"("Boolean"=w565, "Name"="KinectTriggered?") -> ()  [unwired: 8 in, 2 out]
      }
    }
  }
